vi "Temperature Controller.vi"(8 "error in (no error)":errorcluster, 11 "Temperature Controller in":refnum<class "Temperature Controller.lvclass">) -> (0 "error out":errorcluster, 3 "Temperature Controller out":refnum<class "Temperature Controller.lvclass">)   [LabVIEW 2009, in "Temperature Controller.lvclass"]
uses:
  Temperature Controller.lvclass
  Utility Classes/Readable/Channel Units.ctl
  Global/GPIB Numbers.vi
  Temperature Controller.lvclass/Temperature Controller.ctl
  Utility Classes/Readable/Readable.lvclass
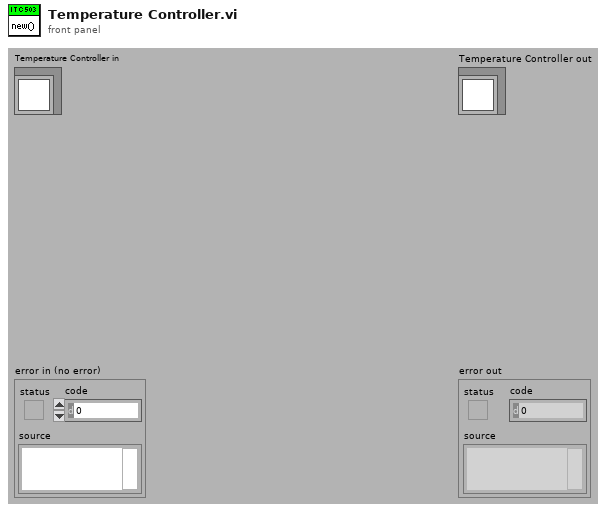
[diagram p1: front panel]
types:
  T1 = typedef "Readable.lvclass/Channel Units.ctl" = string[]
  T2 = typedef "ITCIO.ctl" = cluster{"Address":T3, "Version":T4, "Ch 1 dec places":i16, "Ch 2 dec places":i16, "Ch 3 dec places":i16, "Ch1 Name":string, "Ch2 Name":string, "Ch3 Name":string}
  T3 = typedef "OxfordAddress.ctl" = cluster{"Com Port":i32, "ISOBUS Address":i32, "GPIB Address":i16, "Communication":enum16{"RS232", "ISOBUS", "GPIB", "Gateway"}}
  T4 = typedef "ITCVersion.ctl" = enum16{"ITC502", "ITC503", "ITC601"}
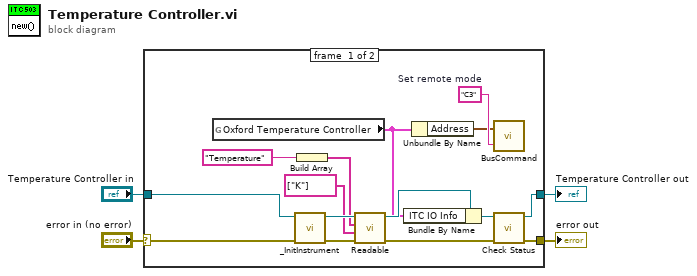
[diagram p0: block diagram]
diagram:
  n1 = case shown="No Error" "error in (no error)" {
    selector: "error in (no error)" -> [w14 w21]
    tunnel: [w16 w21] -> w3
    tunnel: [w17 w20] -> w1
    tunnel: "Temperature Controller in" -> [w19 w20]
    frame #0 {
      w7 = "C3"  # Set remote mode
      n2 = global read "GPIB Numbers.vi" "Oxford Temperature Controller"() -> (w5:T2)
      n3 = call-dynamic "_InitInstrument.vi"("error in (no error)"=w14, "Instrument in"=w19) -> ("error out"=w12:errorcluster, "Instrument out"=w15:refnum<class "Temperature Controller.lvclass">)  [unwired: 8 in]
      n4 = Build Array("Temperature") -> (w8:string[])
      n5 = call "Readable.vi"("error in (no error)"=w12, "Channel Units"=T1 ["K"], "Channel Names"=w8, "Readable in"=w15) -> ("error out"=w11:errorcluster, "Readable out"=w13:refnum<class "Temperature Controller.lvclass">)  [unwired: 6 in]
      n6 = Bundle By Name(cluster=w13, "ITC IO Info"=w5) -> (w18:refnum<class "Temperature Controller.lvclass">)
      n7 = Unbundle By Name(w5) -> ("Address"=w6:T3)
      n8 = call "BusCommand.vi"("Command"=w7, "Instrument address (in)"=w6) -> ()  [unwired: 2 out]
      n9 = call-dynamic "Check Status.vi"("error in (no error)"=w11, "Temperature Controller in"=w18) -> ("error out"=w16:errorcluster, "Temperature Controller out"=w17:refnum<class "Temperature Controller.lvclass">)  [unwired: 6 in, 2 out]
    }
    frame #1 {
    }
  }
  "error out" <- w3
  "Temperature Controller out" <- w1
